vi "FGGA_Dry_Conditions.vi"(0 "CH4_Dry":dbl, 7 "Pressure":dbl, 11 "CO2_Dry":dbl) -> (4 "CH4_Dry_TCP":string, 6 "CH4_Dry_UDP":string, 10 "CO2_Dry_TCP":string, 15 "CO2_Dry_UDP":string)   [LabVIEW 2014]
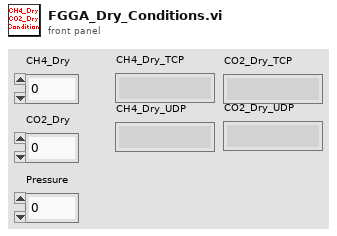
[diagram p1: front panel]
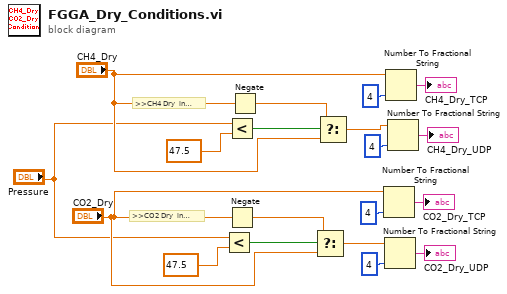
[diagram p0: block diagram]
diagram:
  # ">>CO2 Dry  in ppm>>"
  # ">>CH4 Dry  in ppb>>"
  n1 = Less?(x="Pressure", y=47.5) -> (x < y?=w12:bool)
  n2 = Less?(x="Pressure", y=47.5) -> (x < y?=w17:bool)
  n3 = Negate(x="CO2_Dry") -> (-x=w11:dbl)
  n4 = Negate(x="CH4_Dry") -> (-x=w16:dbl)
  n5 = Select(t=w11, s=w12, f="CO2_Dry") -> (s? t:f=w10:dbl)
  n6 = Select(t=w16, s=w17, f="CH4_Dry") -> (s? t:f=w15:dbl)
  n7 = Number To Fractional String(number="CO2_Dry", precision (6)=i16 4) -> (F-format string=→"CO2_Dry_TCP":string)  [unwired: 2 in]
  n8 = Number To Fractional String(number=w10, precision (6)=i16 4) -> (F-format string=→"CO2_Dry_UDP":string)  [unwired: 2 in]
  n9 = Number To Fractional String(number="CH4_Dry", precision (6)=i16 4) -> (F-format string=→"CH4_Dry_TCP":string)  [unwired: 2 in]
  n10 = Number To Fractional String(number=w15, precision (6)=i16 4) -> (F-format string=→"CH4_Dry_UDP":string)  [unwired: 2 in]
